vi "AddSteppedCurrent.vi"(0 "deviceName":string, 1 "endCurrent":sgl, 2 "stepSize":sgl, 3 "approxMaxVoltage":sgl=inf, 5 "channel":u8, 7 "repeats":u16=1, 9 "startCurrent":sgl, 11 "error in (no error)":errorcluster, 12 "samplingInterval":sgl, 13 "stepDuration":sgl, 14 "approxMinVoltage":sgl=-inf) -> (15 "error out":errorcluster)   [LabVIEW 2018]
doc: "EXPORT void AisAddSteppedCurrent(const char* deviceName, uint8_t channel, uint16_t repeats, float startCurrent, float endCurrent, float samplingInterval, float stepSize, float stepDuration, float approxMaxVoltage, float approxMinVoltage);"
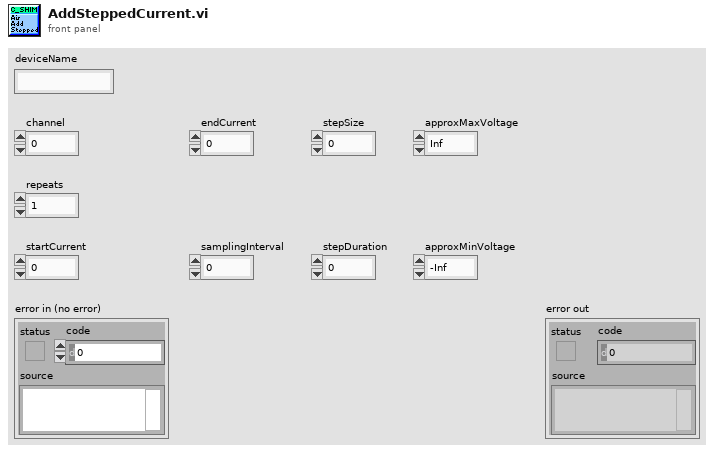
[diagram p1: front panel]
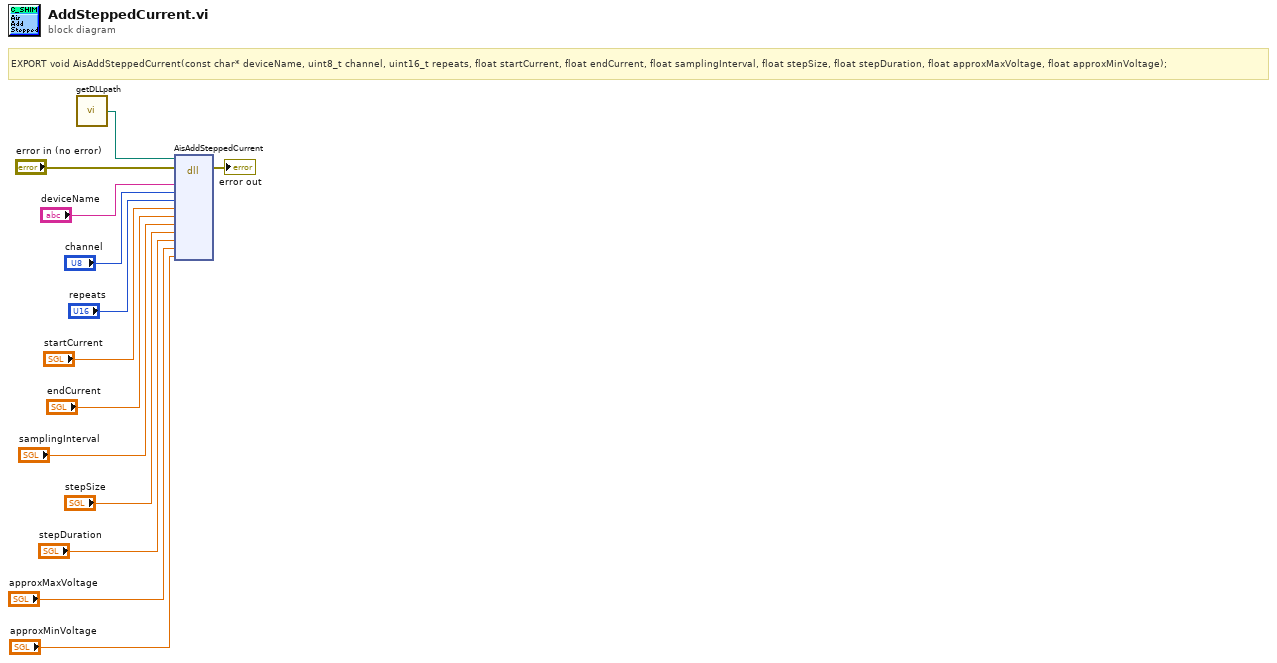
[diagram p0: block diagram]
diagram:
  # "EXPORT void AisAddSteppedCurrent(const char* deviceName, uint8_t channel, uint16_t repeats, float startCurrent, float endCurrent, float samplingInterval, float stepSize, float stepDuration, float approxMaxVoltage, float approxMinVoltage);"
  n1 = call "getDLLpath.vi"() -> ("DLL_Path"=w1:path)
  n2 = dll-call lib="?" fn="AisAddSteppedCurrent"(path in=w1, error in="error in (no error)", "deviceName"="deviceName", "channel"="channel", "repeats"="repeats", "startCurrent"="startCurrent", "endCurrent"="endCurrent", "samplingInterval"="samplingInterval", "stepSize"="stepSize", "stepDuration"="stepDuration", "approxMaxVoltage"="approxMaxVoltage", "approxMinVoltage"="approxMinVoltage") -> (error out=→"error out":errorcluster)  [unwired: 12 in, 1 out]
